vi "Convert Data.vi"(8 "error in (no error)":errorcluster, 11 "tags in":refnum<class "NI Skyline Tag.lvclass">[](array[class])) -> (0 "error out":errorcluster, 3 "table of tag data":string[][](array[string]))   [LabVIEW 2020, in "FlexLoggerTagHelpers.lvlib"]
doc: "Indexes through the array of data, converting each element to a string based on it's data type."
uses:
  FlexLoggerTagHelpers.lvlib
  <vilib>/Skyline/Tag/Wrapper/Wrapper_class/NI Skyline Tag.lvclass
  <vilib>/Skyline/Tag/Wrapper/Wrapper_class/NI Skyline Tag.lvclass/NI Skyline Tag.ctl
  <vilib>/Skyline/Tag/Shared/typedefs/Aggregates Double.ctl
  <vilib>/Skyline/Tag/Wrapper/Wrapper_class/Read Tag Path.vi
  <vilib>/Skyline/Tag/Wrapper/Wrapper_class/Read Tag (U64).vi
  <vilib>/Skyline/Tag/Wrapper/Wrapper_class/Read Tag (Timestamp).vi
  <vilib>/Skyline/Tag/Wrapper/Wrapper_class/Read Tag (String).vi
  <vilib>/Skyline/Tag/Wrapper/Wrapper_class/Read Tag (I32).vi
  <vilib>/Skyline/Tag/Wrapper/Wrapper_class/Read Tag (Boolean).vi
  <vilib>/Skyline/Tag/Wrapper/Wrapper_class/Read Tag (DBL).vi
  <vilib>/Skyline/Tag/Shared/NI Skyline Tag.lvlib
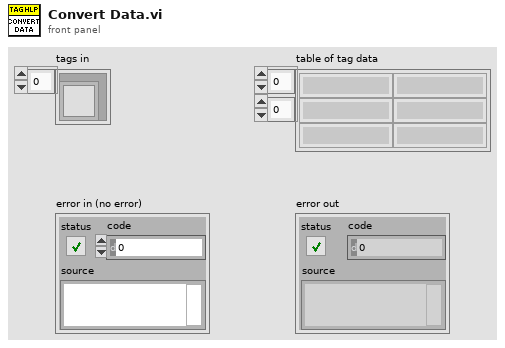
[diagram p1: front panel]
types:
  T1 = typedef "NI Skyline Tag.lvlib/Aggregates Double.ctl" = cluster{"Count":i32, "Max":dbl, "Min":dbl, "Mean":dbl}
  T2 = typedef "NI Skyline Tag.lvlib/DataType.ctl" = enum32{"Double", "I32", "String", "Boolean", "U64", "Timestamp"}
  T3 = typedef "NI Skyline Tag.lvlib/Aggregates Int.ctl" = cluster{"Count":i32, "Max":i32, "Min":i32, "Mean":dbl}
  T4 = typedef "NI Skyline Tag.lvlib/Aggregates U64.ctl" = cluster{"Count":i32, "Max":u64, "Min":u64, "Mean":dbl}
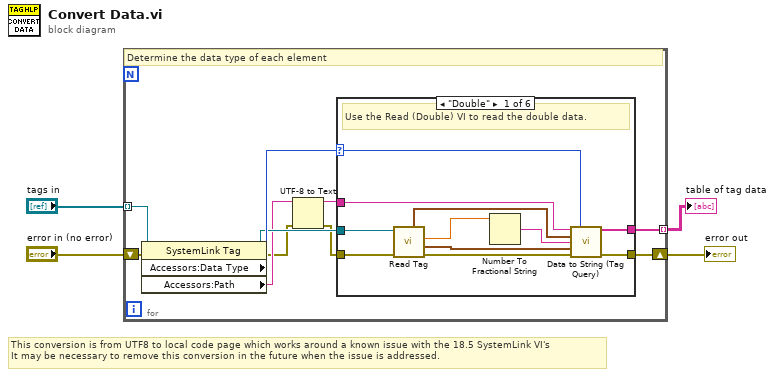
[diagram p0: block diagram]
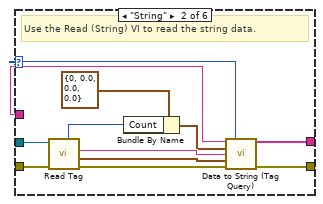
[diagram p2: hidden frame]
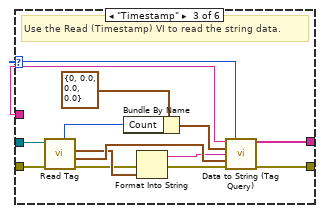
[diagram p3: hidden frame]
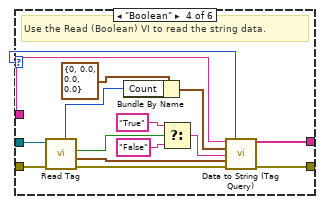
[diagram p4: hidden frame]
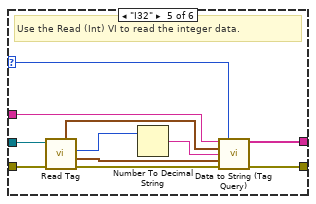
[diagram p5: hidden frame]
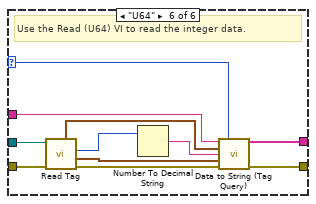
[diagram p6: hidden frame]
diagram:
  # "This conversion is from UTF8 to local code page which works around a known issue with the 18.5 SystemLink VI's\nIt may be necessary to remove this conversion in the future when the issue is addressed."
  n1 = for {
    tunnel: "tags in" -> [w12] mode=indexing
    tunnel: [w14] -> w3 mode=indexing
    shift-right: [w13] -> w4
    shift-left: "error in (no error)" -> [w9]
    # "Determine the data type of each element"
    n2 = property class="SystemLink Tag"(reference=w12, error in=w9) -> (reference out=w10:refnum<class "NI Skyline Tag.lvclass">, error out=w6:errorcluster, "Accessors:Data Type"=w11:T2, "Accessors:Path"=w8:string)
    n3 = UTF-8 to Text(8:w6, 11:w8) -> (0:w5:errorcluster, 3:w7:string)  [unwired: 1 in]
    n4 = case shown="\"Double\"" w11 {
      selector: w11 -> [w18 w33 w48 w63 w74 w85]
      tunnel: w10 -> [w16 w37 w51 w66 w77 w88]
      tunnel: w5 -> [w15 w36 w50 w65 w76 w87]
      tunnel: [w22 w30 w46 w60 w71 w82] -> w13
      tunnel: [w24 w32 w47 w62 w70 w81] -> w14
      tunnel: w7 -> [w17 w29 w45 w59 w67 w78]
      frame "Double" {
        # "Use the Read (Double) VI to read the double data."
        n5 = call-poly <vilib>:"Read Tag.vi"("error in (no error)"=w15, "tag in"=w16) -> ("error out"=w23:errorcluster, "time stamp"=w21:timestamp, "value"=w25:dbl, "Aggregate Values"=w19:T1)  [unwired: 5 in, 1 out]
        n6 = Number To Fractional String(number=w25) -> (F-format string=w20:string)  [unwired: 3 in]
        n7 = call "Data to String (Tag Query).vi"("tag path"=w17, "data type"=w18, "aggregate values"=w19, "current value"=w20, "time stamp"=w21, "error in (no error)"=w23) -> ("tag string array"=w24:string[], "error out"=w22:errorcluster)  [unwired: 8 in]
      }
      frame "String" {
        # "Use the Read (String) VI to read the string data."
        n8 = call-poly <vilib>:"Read Tag.vi"("error in (no error)"=w36, "tag in"=w37) -> ("error out"=w31:errorcluster, "time stamp"=w35:timestamp, "value"=w34:string, "count"=w27:i32)  [unwired: 5 in, 1 out]
        n9 = Bundle By Name(cluster=T1 {"Count"=0, "Max"=0.0, "Min"=0.0, "Mean"=0.0} ("Aggregate Values"), "Count"=w27) -> (w26:T1)
        n10 = call "Data to String (Tag Query).vi"("tag path"=w29, "data type"=w33, "aggregate values"=w26, "current value"=w34, "time stamp"=w35, "error in (no error)"=w31) -> ("tag string array"=w32:string[], "error out"=w30:errorcluster)  [unwired: 8 in]
      }
      frame "Timestamp" {
        # "Use the Read (Timestamp) VI to read the string data."
        n11 = call-poly <vilib>:"Read Tag.vi"("error in (no error)"=w50, "tag in"=w51) -> ("error out"=w39:errorcluster, "time stamp"=w49:timestamp, "value"=w40:timestamp, "count"=w43:i32)  [unwired: 5 in, 1 out]
        n12 = Bundle By Name(cluster=T1 {"Count"=0, "Max"=0.0, "Min"=0.0, "Mean"=0.0} ("Aggregate Values"), "Count"=w43) -> (w42:T1)
        n13 = Format Into String(error in=w39, w40) -> (resulting string=w41:string, error out=w38:errorcluster)  [unwired: 2 in]
        n14 = call "Data to String (Tag Query).vi"("tag path"=w45, "data type"=w48, "aggregate values"=w42, "current value"=w41, "time stamp"=w49, "error in (no error)"=w38) -> ("tag string array"=w47:string[], "error out"=w46:errorcluster)  [unwired: 8 in]
      }
      frame "Boolean" {
        # "Use the Read (Boolean) VI to read the string data."
        n15 = call-poly <vilib>:"Read Tag.vi"("error in (no error)"=w65, "tag in"=w66) -> ("error out"=w61:errorcluster, "time stamp"=w64:timestamp, "value"=w55:bool, "count"=w57:i32)  [unwired: 5 in, 1 out]
        n16 = Bundle By Name(cluster=T1 {"Count"=0, "Max"=0.0, "Min"=0.0, "Mean"=0.0} ("Aggregate Values"), "Count"=w57) -> (w56:T1)
        n17 = Select(t="True", s=w55, f="False") -> (s? t:f=w52:string)
        n18 = call "Data to String (Tag Query).vi"("tag path"=w59, "data type"=w63, "aggregate values"=w56, "current value"=w52, "time stamp"=w64, "error in (no error)"=w61) -> ("tag string array"=w62:string[], "error out"=w60:errorcluster)  [unwired: 8 in]
      }
      frame "I32" {
        # "Use the Read (Int) VI to read the integer data."
        n19 = call-poly <vilib>:"Read Tag.vi"("error in (no error)"=w76, "tag in"=w77) -> ("error out"=w68:errorcluster, "time stamp"=w69:timestamp, "value"=w75:i32, "Aggregate Values"=w73:T3)  [unwired: 5 in, 1 out]
        n20 = Number To Decimal String(number=w75) -> (decimal integer string=w72:string)  [unwired: 1 in]
        n21 = call "Data to String (Tag Query).vi"("tag path"=w67, "data type"=w74, "aggregate values"=w73, "current value"=w72, "time stamp"=w69, "error in (no error)"=w68) -> ("tag string array"=w70:string[], "error out"=w71:errorcluster)  [unwired: 8 in]
      }
      frame "U64" {
        # "Use the Read (U64) VI to read the integer data."
        n22 = call-poly <vilib>:"Read Tag.vi"("error in (no error)"=w87, "tag in"=w88) -> ("error out"=w79:errorcluster, "time stamp"=w80:timestamp, "value"=w86:u64, "Aggregate Values"=w84:T4)  [unwired: 5 in, 1 out]
        n23 = Number To Decimal String(number=w86) -> (decimal integer string=w83:string)  [unwired: 1 in]
        n24 = call "Data to String (Tag Query).vi"("tag path"=w78, "data type"=w85, "aggregate values"=w84, "current value"=w83, "time stamp"=w80, "error in (no error)"=w79) -> ("tag string array"=w81:string[], "error out"=w82:errorcluster)  [unwired: 8 in]
      }
    }
  }
  "error out" <- w4
  "table of tag data" <- w3
